vi "Test Subpanels.vi"() -> ()   [LabVIEW 2012]
panel:
  in  "Boolean":bool
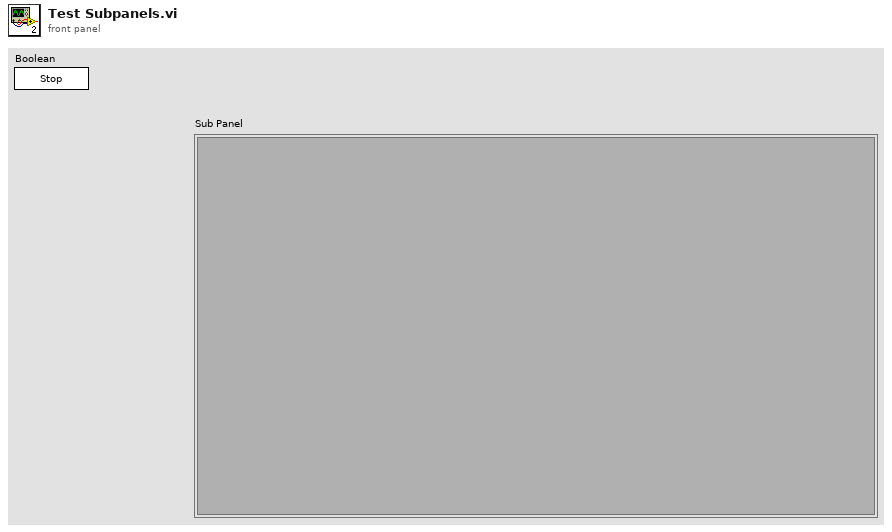
[diagram p1: front panel]
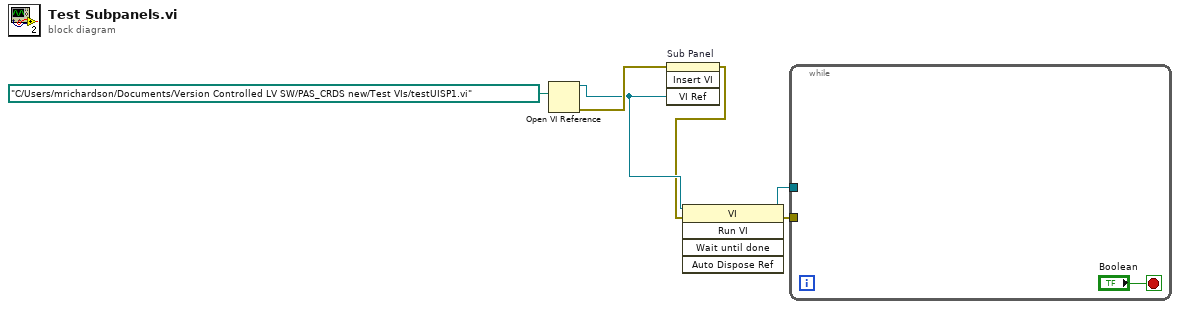
[diagram p0: block diagram]
diagram:
  n1 = Open VI Reference(vi path=path "C:/Users/mrichardson/Documents/Version Controlled LV SW/PAS_CRDS new/Test VIs/testUISP1.vi") -> (vi reference=w4:refnum<vi>, error out=w5:errorcluster)  [unwired: 5 in]
  n2 = invoke on="Sub Panel" class="SubPanel" method="Insert VI"(error in=w5, "VI Ref"=w4) -> (error out=w2:errorcluster)  [unwired: 2 in, 3 out]
  n3 = invoke class="VI" method="Run VI"(reference=w4, error in=w2) -> (reference out=w3:refnum<vi>, error out=w1:errorcluster)  [unwired: 3 in, 3 out]
  n4 = while {
    tunnel: w3 -> [_]
    tunnel: w1 -> [_]
    stop <- "Boolean" stop-if-true
  }
